vi "Pixycam_Read.vi"(8 "error in":errorcluster, 11 "PixySPIDevRef":T1={"DevStatus"={"status"=FALSE, "code"=0, "source"=""}, "Handle"=0, "Controller"=enum."Controller 1", "SPI Bus"=enum."Invalid"}) -> ()   [LabVIEW 2014]
uses:
  <vilib>/Rock Robotics/WPI/SPI/WPI_SPIDevRef.ctl
  <vilib>/Rock Robotics/SystemInterfaces/Typedef/FPGA_TypedefDigitalModule.ctl
  <vilib>/Rock Robotics/SystemInterfaces/spilib/spi_bus.ctl
panel:
  out "Block Sync":u16 format="%x"
  out "Checksum OK":bool
  out "Height":u16
  out "Width":u16
  out "Y Center":u16
  out "X Center":u16
  out "Signature":u16
  out "Checksum":u16
  out "Object Sync":u16 format="%x"
  out "Recieved Data":u16[](array[numeric])
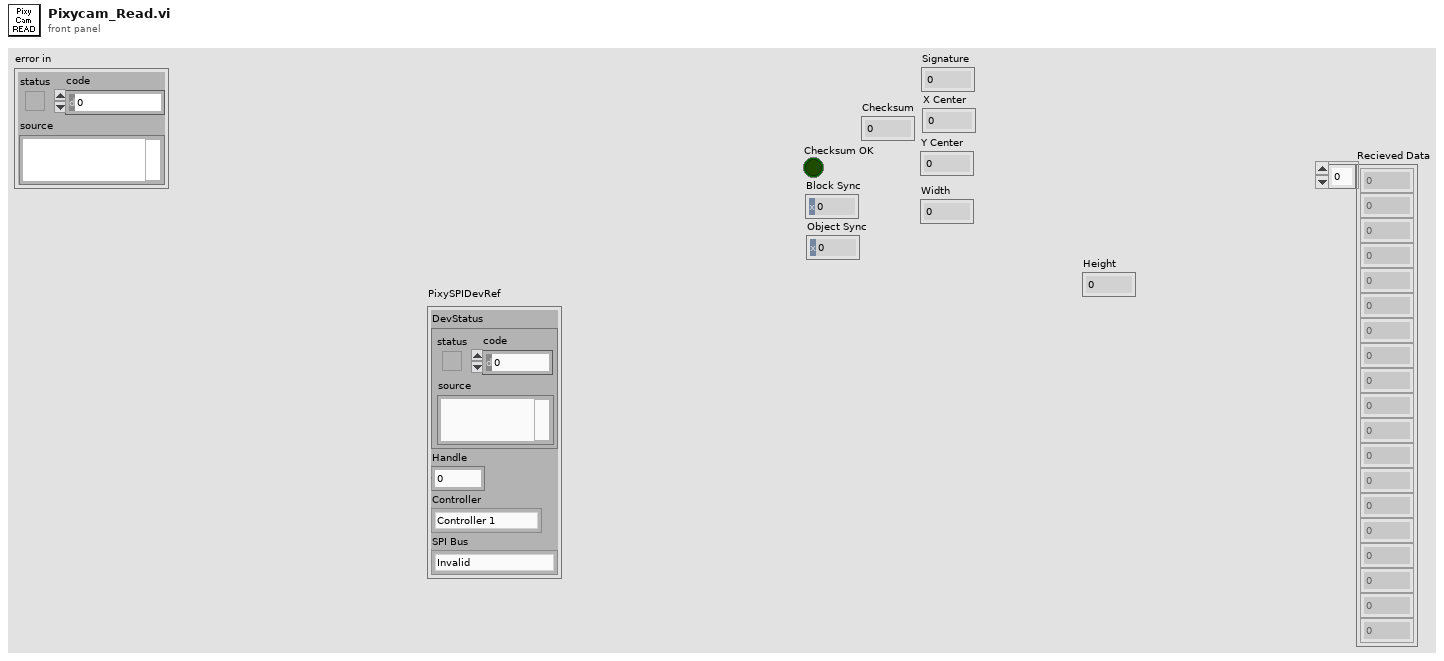
[diagram p1: front panel]
types:
  T1 = typedef "WPI_SPIDevRef.ctl" = cluster{"DevStatus":errorcluster, "Handle":i32, "Controller":T2, "SPI Bus":T3}
  T2 = typedef "FPGA_TypedefDigitalModule.ctl" = enum16{"Controller 1"}
  T3 = typedef "spi_bus.ctl" = enum16{"SPI On-Board, CS0", "SPI On-Board, CS1", "SPI On-Board, CS2", "SPI On-Board, CS3", "SPI MXP", "Invalid"}
  T4 = enum16{"big-endian, network order", "native, host order", "little-endian"}
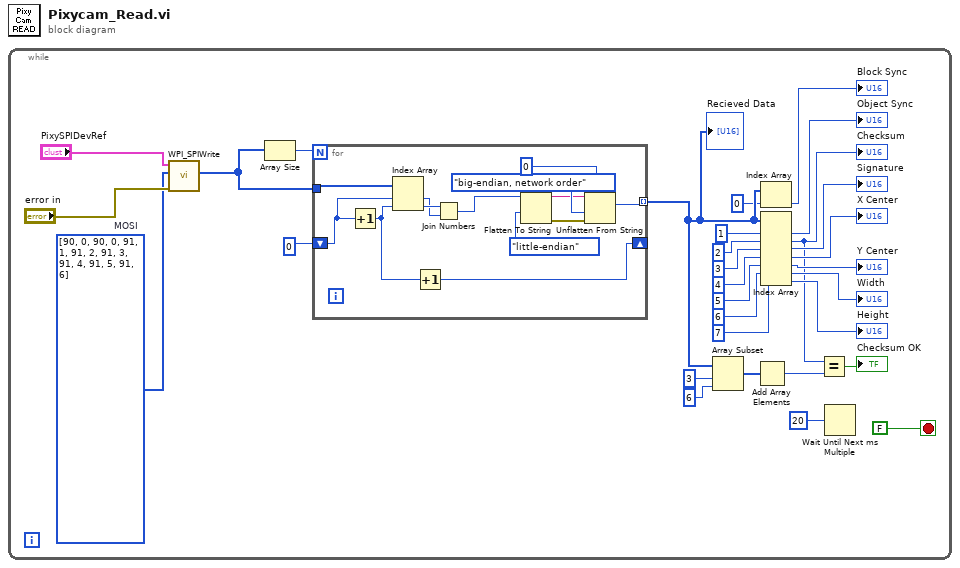
[diagram p0: block diagram]
diagram:
  n1 = while {
    stop <- FALSE stop-if-true
    w2 = u8[] [90, 0, 90, 0, 91, 1, 91, 2, 91, 3, 91, 4, 91, 5, 91, 6]  # MOSI
    n2 = call <vilib>:"WPI_SPIWrite.vi"("error in (no error)"="error in", "Data To Send"=w2, "SPIDevRef"="PixySPIDevRef") -> ("Received Data"=w8:u8[])  [unwired: 6 in, 2 out]
    n3 = Array Size(array=w8) -> (size(s)=w9:i32)
    n4 = for {
      N: w9 -> [_]
      tunnel: w8 -> [w43]
      tunnel: [w36] -> w5 mode=indexing
      shift-right: [w31] -> _
      shift-left: 0 ("index") -> [w33]
      n5 = Increment(x=w33) -> (x+1=w32:i32)
      n6 = Index Array(array=w43, index #1=w33, index #2=w32) -> (element #1=w41:u8, element #2=w42:u8)
      n7 = Increment(x=w32) -> (x+1=w31:i32)
      n8 = Join Numbers(hi=w42, lo=w41) -> ((hi.lo)=w35:u16)
      n9 = Flatten To String(anything=w35, byte order (0:big-endian, network order)=T4."little-endian") -> (data string=w37:string, error out=w40:errorcluster)  [unwired: 2 in, 1 out]
      n10 = Unflatten From String(type=u16 0, binary string=w37, byte order (0:big-endian, network order)=T4."big-endian, network order", error in (no error)=w40) -> (value=w36:u16)  [unwired: 1 in, 2 out]
    }
    "Recieved Data" <- w5
    n11 = Array Subset(array=w5, index=3, length=6) -> (w13:u16[])
    n12 = Add Array Elements(numeric array=w13) -> (sum=w12:u16)
    n13 = Index Array(array=w5, index=0) -> (element=→"Block Sync":u16)
    n14 = Index Array(array=w5, index #1=1 ("index"), index #2=2 ("index"), index #3=3 ("index"), index #4=4 ("index"), index #5=5 ("index"), index #6=6 ("index"), index #7=7 ("index")) -> (element #1=→"Object Sync":u16, element #2=w11:u16, element #3=→"Signature":u16, element #4=→"X Center":u16, element #5=→"Y Center":u16, element #6=→"Width":u16, element #7=→"Height":u16)
    "Checksum" <- w11
    n15 = Equal?(x=w11, y=w12) -> (x = y?=→"Checksum OK":bool)
    n16 = Wait Until Next ms Multiple(millisecond multiple=u32 20) -> ()  [unwired: 1 out]
  }
